vi "emi_Window Set position and seperators.vi"(2 "Section(VI Name)":string, 5 "VI Refnum(This VI)":refnum<vi>, 9 "error in (no error)":errorcluster, 13 "Set Splitters(T)":bool=TRUE) -> (6 "VI Refnum":refnum<vi>, 10 "error out":errorcluster)   [LabVIEW 2011]
doc: "If window position and size in ini file: Set position to last. Else: Senter\nIf window resisable: Set size to last: Else. Leave size alone\nIf splitters(T) = true, and splitters in window and splitters in file, set splitter position.\nTries to trigger window resize.\nIf window wends up outside screen, it gets sentered\n\nStore the window position, and splitters in ini file.\n\nOn error: Tries to senter the window"
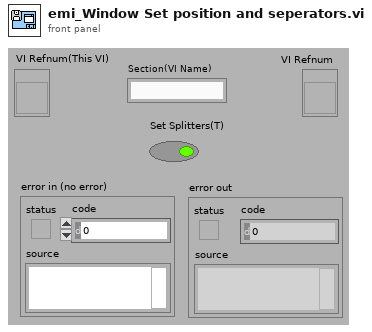
[diagram p1: front panel]
types:
  T1 = enum32{"Invalid", "Standard", "Closed", "Hidden", "Minimized", "Maximized"}
  T2 = typedef "LVRectTypeDef.ctl" = cluster{"left":i16, "top":i16, "right":i16, "bottom":i16}
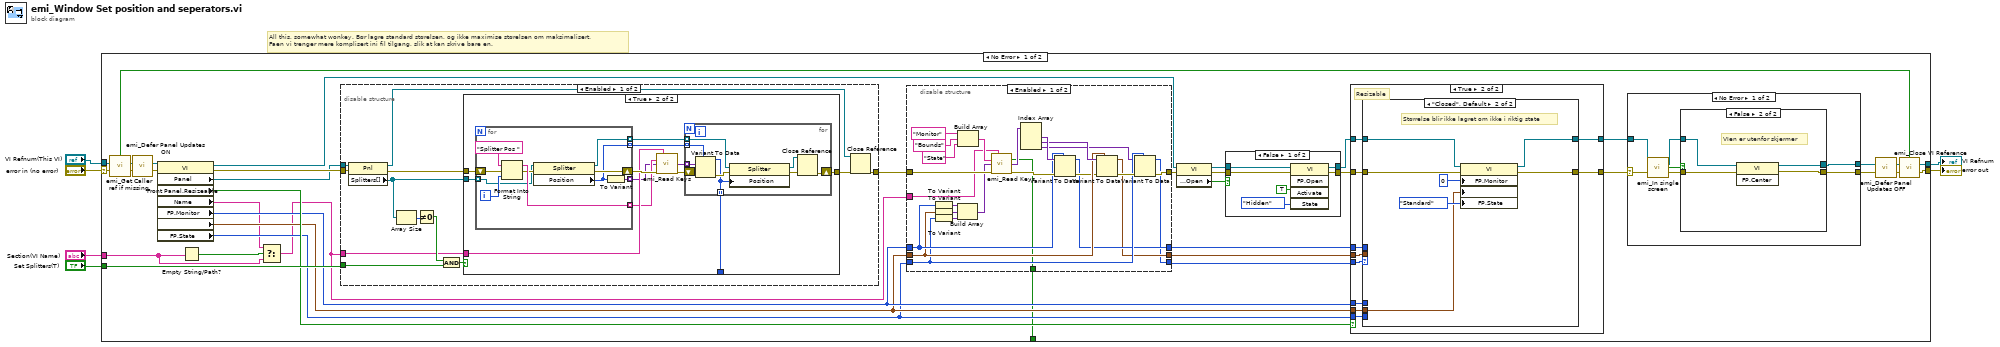
[diagram p0: block diagram]
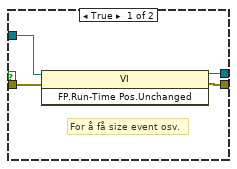
[diagram p3: hidden frame]
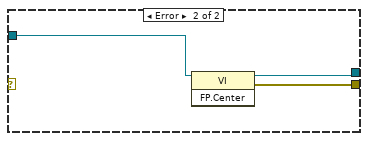
[diagram p4: hidden frame]
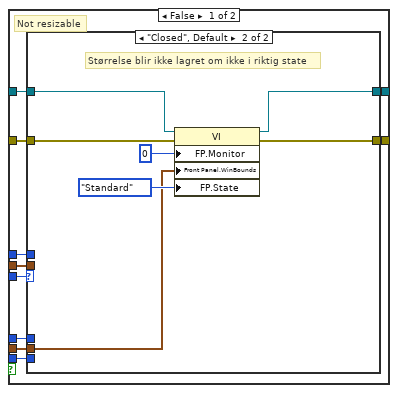
[diagram p5: hidden frame]
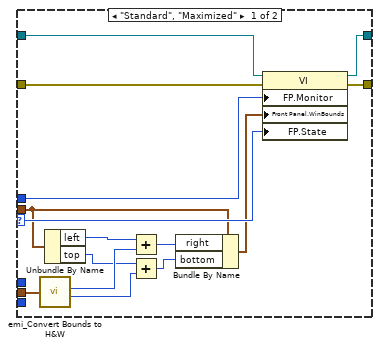
[diagram p6: hidden frame]
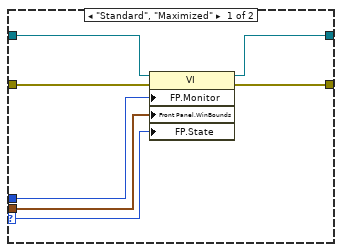
[diagram p7: hidden frame]
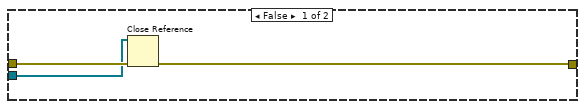
[diagram p9: hidden frame]
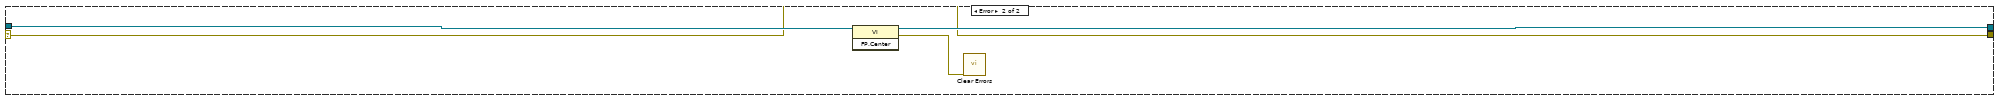
[diagram p11: hidden frame]
diagram:
  # "All this, somewhat wonkey. Bør lagre standard størelsen, og ikke maximise størelsen om maksimalisert.\nFaen vi trenger mere komplisert ini fil tilgang, slik at kan skrive bare en."
  n1 = case shown="No Error" "error in (no error)" {
    selector: "error in (no error)" -> [w42 w200]
    tunnel: "VI Refnum(This VI)" -> [w44 w202]
    tunnel: [w24 w200] -> w5
    tunnel: [w23 w201] -> w4
    tunnel: "Set Splitters(T)" -> [w39 _]
    tunnel: [w20 _] -> _
    tunnel: "Section(VI Name)" -> [w16 _]
    frame No Error {
      n2 = call "emi_Get Caller ref if missing.vi"("VI Refnum(Calling VI)"=w44, "error in (no error)"=w42) -> ("Ref Generated"=w43:bool, "VI Refnum Out"=w28:refnum<vi>, "error out"=w30:errorcluster)  [unwired: 11 in]
      n3 = call "emi_Defer Panel Updates ON.vi"("VI Refnum(This VI)"=w28, "error in (no error)"=w30) -> ("VI Refnum Out"=w27:refnum<vi>, "error out"=w29:errorcluster)  [unwired: 12 in]
      n4 = property class="VI"(reference=w27, error in=w29) -> (reference out=w10:refnum<vi>, error out=w41:errorcluster, "Panel"=w40:refnum<vi>, "Front Panel.Resizeable"=w37:bool, "Name"=w15:string, "FP.Monitor"=w33:u16, "Front Panel.WinBounds"=w32:T2, "FP.State"=w31:T1)
      n5 = Empty String/Path?(string/path=w16) -> (empty?=w17:bool)
      n6 = Select(t=w15, s=w17, f=w16) -> (s? t:f=w14:string)
      n7 = disable-structure shown="Enabled" {
        disable-tunnel: w41 -> [w162 w198]
        disable-tunnel: w40 -> [w161 _]
        disable-tunnel: w39 -> [w157 _]
        disable-tunnel: w14 -> [w155 _]
        disable-tunnel: [w153 w198] -> w38
        frame Enabled {
          n8 = property class="Pnl"(reference=w161, error in=w162) -> (reference out=w163:refnum<vi>, error out=w156:errorcluster, "Splitters[]"=w160:refnum<vi>[])
          n9 = Array Size(array=w160) -> (size(s)=w159:i32)
          n10 = Not Equal To 0?(x=w159) -> (x != 0?=w158:bool)
          n11 = And(x=w158, y=w157) -> (x .and. y?=w152:bool)
          n12 = case shown="True" w152 {
            tunnel: w156 -> [w166 w178]
            tunnel: w160 -> [w165 w177]
            tunnel: w155 -> [_ w175]
            tunnel: [w164 w168] -> w154
            tunnel: [_ w167] -> _
            frame False {
              n13 = Close Reference(reference=w165, error in (no error)=w166) -> (error out=w164:errorcluster)
            }
            frame True {
              n14 = for {
                tunnel: w177 -> [w192] mode=indexing
                tunnel: [w196] -> w174 mode=indexing
                shift-right: [w190] -> w176
                shift-left: w178 -> [w194]
                tunnel: [w191] -> w173 mode=indexing
                tunnel: [w189] -> w170 mode=indexing
                tunnel: [w188] -> w169 mode=indexing
                i -> [w195]
                n15 = Format Into String(initial string="Splitter Pos ", error in=w194, w195) -> (resulting string=w196:string, error out=w193:errorcluster)  [unwired: 1 in]
                n16 = property class="Splitter"(reference=w192, error in=w193) -> (reference out=w189:refnum<vi>, error out=w190:errorcluster, "Position"=w188:i32)
                n17 = To Variant(anything=w188) -> (Variant=w191:variant)
              }
              n18 = call "emi_Read Keys.vi"("Section"=w175, "Key Names"=w174, "Types/Defaults"=w173, "error in (no error)"=w176) -> ("Values"=w171:variant[], "error out"=w172:errorcluster)  [unwired: 9 in, 1 out]
              n19 = for {
                tunnel: w171 -> [w185] mode=indexing
                tunnel: w170 -> [w187] mode=indexing
                tunnel: w169 -> [w184] mode=indexing
                shift-right: [w181] -> w168
                shift-left: w172 -> [w186]
                tunnel: [w179] -> w167 mode=indexing
                n20 = Variant To Data(error in=w186, type=w184, Variant=w185) -> (data=w179:i32, error out=w183:errorcluster)
                n21 = property class="Splitter"(reference=w187, error in=w183, "Position"=w179) -> (reference out=w180:refnum<vi>, error out=w182:errorcluster)
                n22 = Close Reference(reference=w180, error in (no error)=w182) -> (error out=w181:errorcluster)
              }
            }
          }
          n23 = Close Reference(reference=w163, error in (no error)=w154) -> (error out=w153:errorcluster)
        }
        frame Disabled {
        }
      }
      n24 = disable-structure shown="Enabled" {
        disable-tunnel: [w131 _] -> w9
        disable-tunnel: w33 -> [w138 _]
        disable-tunnel: w32 -> [w136 _]
        disable-tunnel: w31 -> [w133 _]
        disable-tunnel: w38 -> [w145 _]
        disable-tunnel: w14 -> [w142 _]
        disable-tunnel: [w130 _] -> w36
        disable-tunnel: [w129 _] -> w35
        disable-tunnel: [w128 _] -> w34
        disable-tunnel: [w127 _] -> w20
        frame Enabled {
          n25 = To Variant(anything=w138) -> (Variant=w148:variant)
          n26 = To Variant(anything=w136) -> (Variant=w147:variant)
          n27 = To Variant(anything=w133) -> (Variant=w146:variant)
          n28 = Build Array(w148, w147, w146) -> (w143:variant[])
          n29 = Build Array("Monitor" ("Name"), "Bounds" ("Name"), "State" ("element")) -> (w144:string[])
          n30 = call "emi_Read Keys.vi"("Section"=w142, "Key Names"=w144, "Types/Defaults"=w143, "error in (no error)"=w145) -> ("file created?"=w127:bool, "Values"=w141:variant[], "error out"=w140:errorcluster)  [unwired: 9 in]
          n31 = Index Array(array=w141) -> (element #1=w139:variant, element #2=w137:variant, element #3=w132:variant)  [unwired: 3 in]
          n32 = Variant To Data(error in=w140, type=w138, Variant=w139) -> (data=w130:u16, error out=w135:errorcluster)
          n33 = Variant To Data(error in=w135, type=w136, Variant=w137) -> (data=w129:T2, error out=w134:errorcluster)
          n34 = Variant To Data(error in=w134, type=w133, Variant=w132) -> (data=w128:T1, error out=w131:errorcluster)
        }
        frame Disabled {
        }
      }
      n35 = property class="VI"(reference=w10, error in=w9) -> (reference out=w13:refnum<vi>, error out=w12:errorcluster, "Front Panel.Open"=w11:bool)
      n36 = case shown="False" w11 {
        tunnel: w12 -> [w49 w51]
        tunnel: w13 -> [w50 w52]
        tunnel: [w48 w51] -> w8
        tunnel: [w47 w52] -> w7
        frame False {
          n37 = invoke class="VI" method="FP.Open"(reference=w50, error in=w49, "Activate"=TRUE ("Activate?"), "State"=T1."Hidden") -> (reference out=w47:refnum<vi>, error out=w48:errorcluster)  [unwired: 1 in, 3 out]
        }
        frame True {
        }
      }
      n38 = case shown="True" w37 {
        tunnel: w8 -> [w77 w109]
        tunnel: w36 -> [w78 w110]
        tunnel: w35 -> [w79 w111]
        tunnel: w34 -> [w80 w112]
        tunnel: [w74 w106] -> w18
        tunnel: w7 -> [w76 w108]
        tunnel: [w75 w107] -> w19
        tunnel: w33 -> [w73 w105]
        tunnel: w32 -> [w72 w104]
        tunnel: w31 -> [w71 w103]
        frame False {
          # "Not resizable"
          n39 = case shown="\"Closed\", Default" w80 {
            selector: w80 -> [w91 _]
            tunnel: w79 -> [w88 _]
            tunnel: w78 -> [w92 _]
            tunnel: w77 -> [w95 w102]
            tunnel: w76 -> [w81 w100]
            tunnel: [w93 w99] -> w75
            tunnel: [w94 w101] -> w74
            tunnel: w73 -> [_ _]
            tunnel: w72 -> [w90 w97]
            tunnel: w71 -> [_ _]
            frame "Standard", "Maximized" {
              n40 = call "emi_Convert Bounds to H&W.vi"("Bounds"=w90) -> ("Width"=w86:i32, "Height"=w83:i32)  [unwired: 6 in]
              n41 = Unbundle By Name(w88) -> ("left"=w87:i16, "top"=w84:i16)
              n42 = Add(x=w87, y=w86) -> (x+y=w85:i32)
              n43 = Add(x=w84, y=w83) -> (x+y=w82:i32)
              n44 = Bundle By Name(cluster=w88, "right"=w85, "bottom"=w82) -> (w89:T2)
              n45 = property class="VI"(reference=w81, error in=w95, "FP.Monitor"=w92, "Front Panel.WinBounds"=w89, "FP.State"=w91) -> (reference out=w93:refnum<vi>, error out=w94:errorcluster)
            }
            frame "Closed", Default {
              # "Størrelse blir ikke lagret om ikke i riktig state"
              n46 = property class="VI"(reference=w100, error in=w102, "FP.Monitor"=u16 0 ("Front Panel Window:Monitor"), "Front Panel.WinBounds"=w97, "FP.State"=T1."Standard" ("Front Panel Window:State")) -> (reference out=w99:refnum<vi>, error out=w101:errorcluster)
            }
          }
        }
        frame True {
          # "Resizable"
          n47 = case shown="\"Closed\", Default" w112 {
            selector: w112 -> [w113 _]
            tunnel: w111 -> [w114 _]
            tunnel: w110 -> [w115 _]
            tunnel: w109 -> [w119 w126]
            tunnel: w108 -> [w117 w124]
            tunnel: [w116 w123] -> w107
            tunnel: [w118 w125] -> w106
            tunnel: w105 -> [_ _]
            tunnel: w104 -> [_ w121]
            tunnel: w103 -> [_ _]
            frame "Standard", "Maximized" {
              n48 = property class="VI"(reference=w117, error in=w119, "FP.Monitor"=w115, "Front Panel.WinBounds"=w114, "FP.State"=w113) -> (reference out=w116:refnum<vi>, error out=w118:errorcluster)
            }
            frame "Closed", Default {
              # "Størrelse blir ikke lagret om ikke i riktig state"
              n49 = property class="VI"(reference=w124, error in=w126, "FP.Monitor"=u16 0 ("Front Panel Window:Monitor"), "Front Panel.WinBounds"=w121, "FP.State"=T1."Standard" ("Front Panel Window:State")) -> (reference out=w123:refnum<vi>, error out=w125:errorcluster)
            }
          }
        }
      }
      n50 = case shown="No Error" w18 {
        selector: w18 -> [w53 _]
        tunnel: [w59 w70] -> w22
        tunnel: [w58 w69] -> w21
        tunnel: w19 -> [w57 w68]
        frame No Error {
          n51 = call "emi_In single screen.vi"("VI Refnum(This vi)"=w57, "error in (no error)"=w53) -> ("VI Refnum"=w56:refnum<vi>, "Window in screen"=w54:bool, "error out"=w55:errorcluster)  [unwired: 11 in]
          n52 = case shown="False" w54 {
            tunnel: [w63 w67] -> w59
            tunnel: [w62 w66] -> w58
            tunnel: w56 -> [w61 w65]
            tunnel: w55 -> [w60 w64]
            frame True {
              # "For å få size event osv."
              n53 = invoke class="VI" method="FP.Run-Time Pos.Unchanged"(reference=w61, error in=w60) -> (reference out=w62:refnum<vi>, error out=w63:errorcluster)  [unwired: 1 in, 1 out]
            }
            frame False {
              # "VIen er utenfor skjermer"
              n54 = invoke class="VI" method="FP.Center"(reference=w65, error in=w64) -> (reference out=w66:refnum<vi>, error out=w67:errorcluster)  [unwired: 1 in, 1 out]
            }
          }
        }
        frame Error {
          n55 = invoke class="VI" method="FP.Center"(reference=w68) -> (reference out=w69:refnum<vi>, error out=w70:errorcluster)  [unwired: 2 in, 1 out]
        }
      }
      n56 = call "emi_Defer Panel Updates OFF.vi"("VI Refnum(This VI)"=w21, "error in (no error)"=w22) -> ("VI Refnum Out"=w25:refnum<vi>, "error out"=w26:errorcluster)  [unwired: 12 in]
      n57 = call "emi_Close VI Reference.vi"("Close ref?(T)"=w43, "VI Refnum"=w25, "error in (no error)"=w26) -> ("VI Refnum Out"=w23:refnum<vi>, "error out"=w24:errorcluster)  [unwired: 11 in]
    }
    frame Error {
      n58 = invoke class="VI" method="FP.Center"(reference=w202) -> (reference out=w201:refnum<vi>, error out=w199:errorcluster)  [unwired: 2 in, 1 out]
      n59 = call <vilib>:"Clear Errors.vi"("error in (no error)"=w199) -> ()  [unwired: 6 in, 1 out]
    }
  }
  "error out" <- w5
  "VI Refnum" <- w4
